vi "Error handling.vi"(8 "error in":errorcluster, 10 "User defined error array":T1(array[cluster]), 11 "VI reference":refnum<vi>) -> (0 "error IO":errorcluster, 3 "Error out":string)   [LabVIEW 2015]
uses:
  <userlib>/_OpenG.lib/array/array.llb/Empty 1D Array (Variant)__ogtk.vi
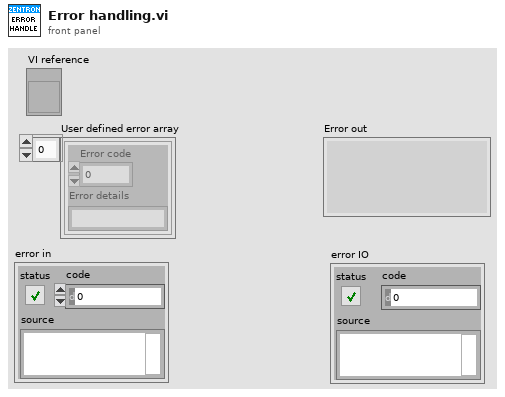
[diagram p1: front panel]
types:
  T1 = cluster{"Error code":i32, "Error details":string}[]
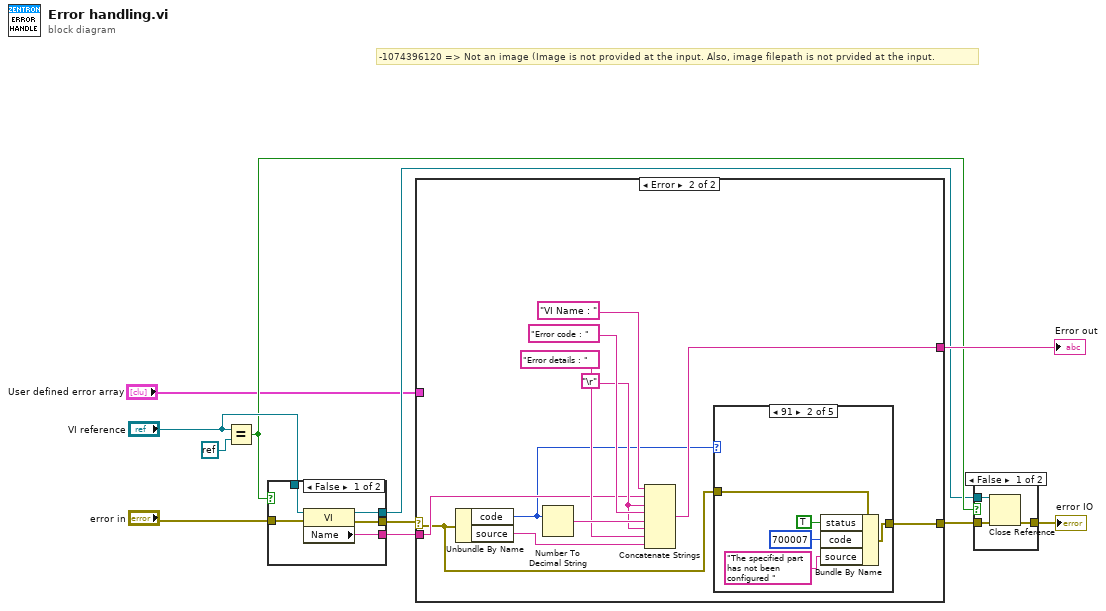
[diagram p0: block diagram]
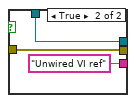
[diagram p3: hidden frame]
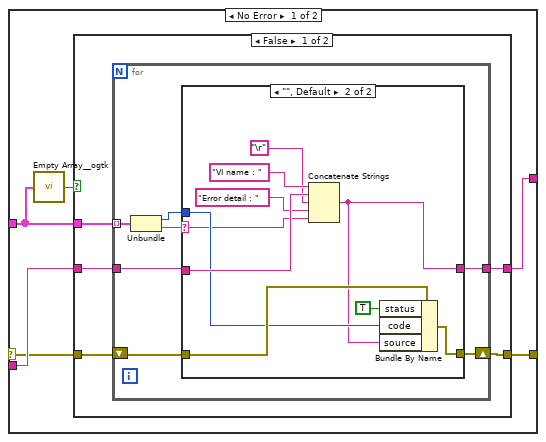
[diagram p4: hidden frame]
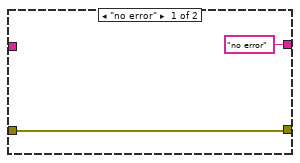
[diagram p5: hidden frame]
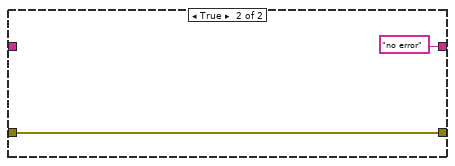
[diagram p6: hidden frame]
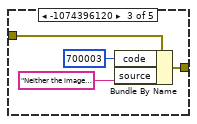
[diagram p8: hidden frame]
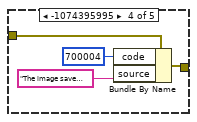
[diagram p9: hidden frame]
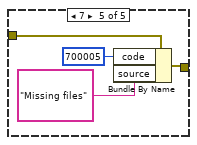
[diagram p10: hidden frame]
diagram:
  # "-1074396120 => Not an image (Image is not provided at the input. Also, image filepath is not prvided at the input."
  n1 = Equal?(x="VI reference", y=refnum<k0> refnum) -> (x = y?=w4:bool)
  n2 = case shown="False" w4 {
    tunnel: "error in" -> [w16 w18]
    tunnel: [w15 "Unwired VI ref" ("Name")] -> w2
    tunnel: [w14 w18] -> w8
    tunnel: "VI reference" -> [w13 w17]
    tunnel: [w12 w17] -> w3
    frame False {
      n3 = property class="VI"(reference=w13, error in=w16) -> (reference out=w12:refnum<vi>, error out=w14:errorcluster, "Name"=w15:string)
    }
    frame True {
    }
  }
  n4 = case shown="Error" w8 {
    selector: w8 -> [w21 w53]
    tunnel: [w24 w56] -> w11
    tunnel: [w20 w52] -> w6
    tunnel: w2 -> [w25 w55]
    tunnel: "User defined error array" -> [w23 _]
    frame No Error {
      n5 = call-poly <userlib>:"Empty Array__ogtk.vi"("Array"=w23) -> ("Empty Array?"=w22:bool)  [unwired: 8 in]
      n6 = case shown="False" w22 {
        tunnel: w25 -> [w30 _]
        tunnel: [w29 "no error"] -> w24
        tunnel: w23 -> [w28 _]
        tunnel: w21 -> [w27 w50]
        tunnel: [w26 w50] -> w20
        frame False {
          n7 = for {
            tunnel: w28 -> [w35] mode=indexing
            tunnel: w30 -> [w37]
            tunnel: [w36] -> w29
            shift-right: [w31] -> w26
            shift-left: w27 -> [w33]
            n8 = Unbundle(w35) -> ("Error code"=w32:i32, "Error details"=w34:string)
            n9 = case shown="\"\", Default" w34 {
              selector: w34 -> [_ w43]
              tunnel: w37 -> [_ w49]
              tunnel: ["no error" w40] -> w36
              tunnel: w33 -> [w38 w45]
              tunnel: w32 -> [_ w44]
              tunnel: [w38 w42] -> w31
              frame "no error" {
              }
              frame "", Default {
                n10 = Concatenate Strings("VI name : ", w49, "\r", "Error detail : ", w43) -> (w40:string)
                n11 = Bundle By Name(cluster=w45, "status"=TRUE, "code"=w44, "source"=w40) -> (w42:errorcluster)
              }
            }
          }
        }
        frame True {
        }
      }
    }
    frame Error {
      w59 = "\r"
      n12 = Unbundle By Name(w53) -> ("code"=w54:i32, "source"=w57:string)
      n13 = Number To Decimal String(number=w54) -> (decimal integer string=w60:string)  [unwired: 1 in]
      n14 = Concatenate Strings("VI Name : " ("string"), w55, w59, "Error code : " ("string"), w60, w59, "Error details : " ("string"), w57) -> (w56:string)
      n15 = case shown="91" w54 {
        tunnel: w53 -> [w63 w68 w72 w73 w77]
        tunnel: [w63 w67 w71 w74 w78] -> w52
        frame 0, Default {
        }
        frame 91 {
          n16 = Bundle By Name(cluster=w68, "status"=TRUE, "code"=700007, "source"="The specified part has not been configured ") -> (w67:errorcluster)
        }
        frame -1074396120 {
          n17 = Bundle By Name(cluster=w72, "code"=700003, "source"="Neither the image nor the image  filepath is provided at the input") -> (w71:errorcluster)
        }
        frame -1074395995 {
          n18 = Bundle By Name(cluster=w73, "code"=700004, "source"="The image save filepath doesn't exist") -> (w74:errorcluster)
        }
        frame 7 {
          n19 = Bundle By Name(cluster=w77, "code"=700005, "source"="Missing files") -> (w78:errorcluster)
        }
      }
    }
  }
  "Error out" <- w11
  n20 = case shown="False" w4 {
    tunnel: w6 -> [w83 w84]
    tunnel: [w82 w84] -> w5
    tunnel: w3 -> [w81 _]
    frame False {
      n21 = Close Reference(reference=w81, error in (no error)=w83) -> (error out=w82:errorcluster)
    }
    frame True {
    }
  }
  "error IO" <- w5
